vi "elvis_dmm_v2.vi"(0 "Device Name":tag="myDAQ3", 1 "Stop":bool=TRUE, 3 "myDAQ Resistance Input Range (Ohms)":sgl(ring)=200.0 items=["200ohm"=200, "2Kohm"=2000, "20Kohm"=20000, "200Kohm"=200000, "2Mohm"=2000000, "20Mohm"=2e+07], 5 "error in":errorcluster) -> (16 "Measurement":dbl, 17 "Overrange":u16(ring) items=["In Range", "+Over", "-Over", "±Over"], 19 "error out":errorcluster)   [LabVIEW 2013]
doc: "Controls the basic Digital Multimeter capabilities of NI ELVIS II."
uses:
  <vilib>/express/NI ELVISmx/misc.llb/ctl_ProductType.ctl
  <vilib>/DAQmx/read.llb/DAQmx Read (Analog 1D Wfm NChan NSamp).vi
  <vilib>/DAQmx/read.llb/DAQmx Read (Analog DBL 1Chan 1Samp).vi
  <vilib>/DAQmx/create/channels.llb/DAQmx Create Channel (AI-Voltage-Basic).vi
  <vilib>/DAQmx/create/channels.llb/DAQmx Create Channel (AI-Voltage-RMS).vi
  <vilib>/DAQmx/create/channels.llb/DAQmx Create Channel (AI-Current-Basic).vi
  <vilib>/DAQmx/create/channels.llb/DAQmx Create Channel (AI-Current-RMS).vi
  <vilib>/DAQmx/create/channels.llb/DAQmx Create Channel (AI-Resistance).vi
  <vilib>/DAQmx/create/channels.llb/DAQmx Create Channel (AO-FuncGen).vi
  <vilib>/DAQmx/configure/timing.llb/DAQmx Timing (Sample Clock).vi
  <vilib>/measure/matone.llb/Extract Single Tone Information 1 Chan.vi
  <vilib>/DAQmx/miscellaneous.llb/DAQmx Fill In Error Info.vi
  <resource>/objmgr/daqmx.rc
  <vilib>/measure/NI_MAPro.lvlib
panel:
  in  "Measurement":T1(ring)=enum."Resistance"
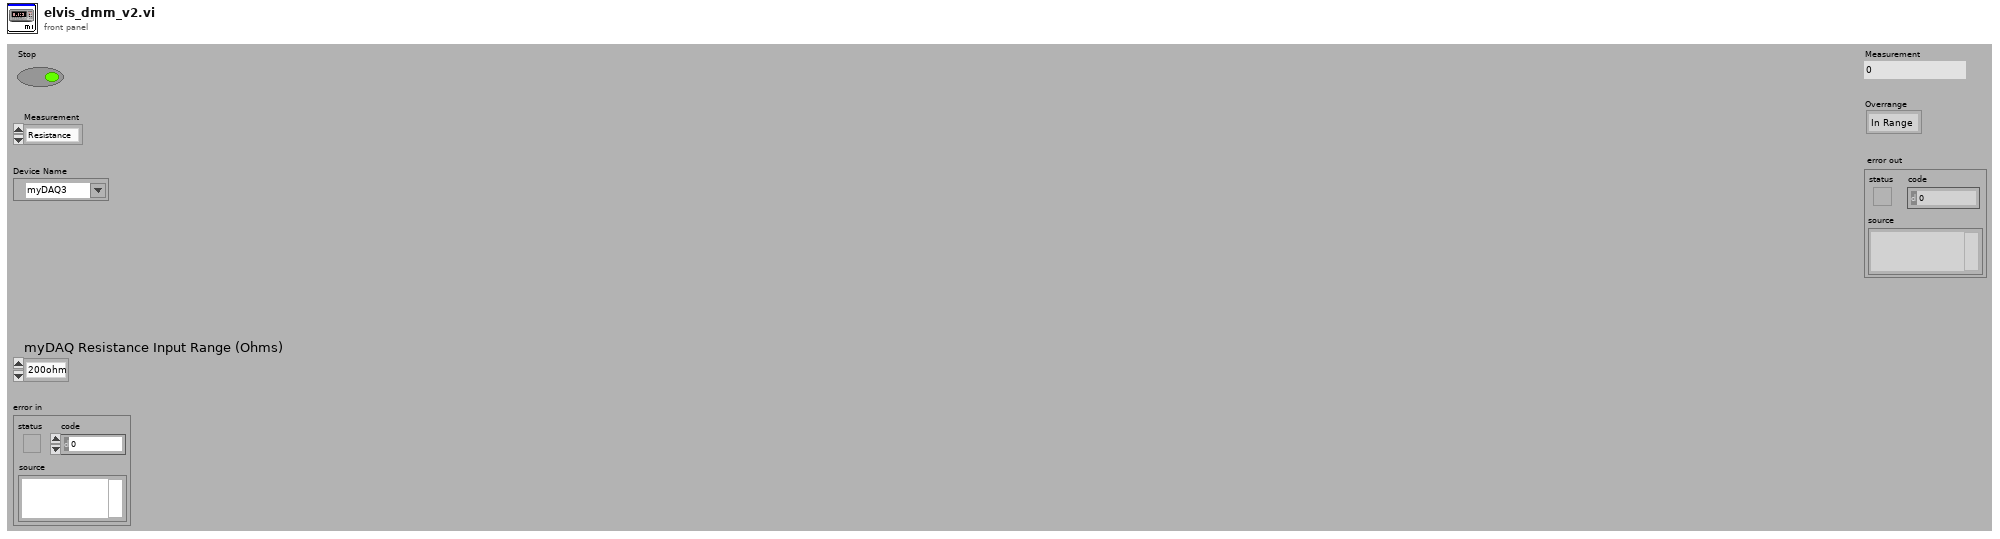
[diagram p1: front panel]
types:
  T1 = enum16{"Volts DC", "Volts AC", "Current DC", "Current AC", "Resistance", "Capacitance", "Inductance", "Diode", "Continuity", "Impedance"}
  T2 = typedef "ctl_ProductType.ctl" = enum16{"NI myDAQ", "NI ELVIS II", "NI ELVIS II+"}
  T3 = cluster{"approx freq. (optional)":dbl, "search (+/- % of Fsampl.)":dbl}
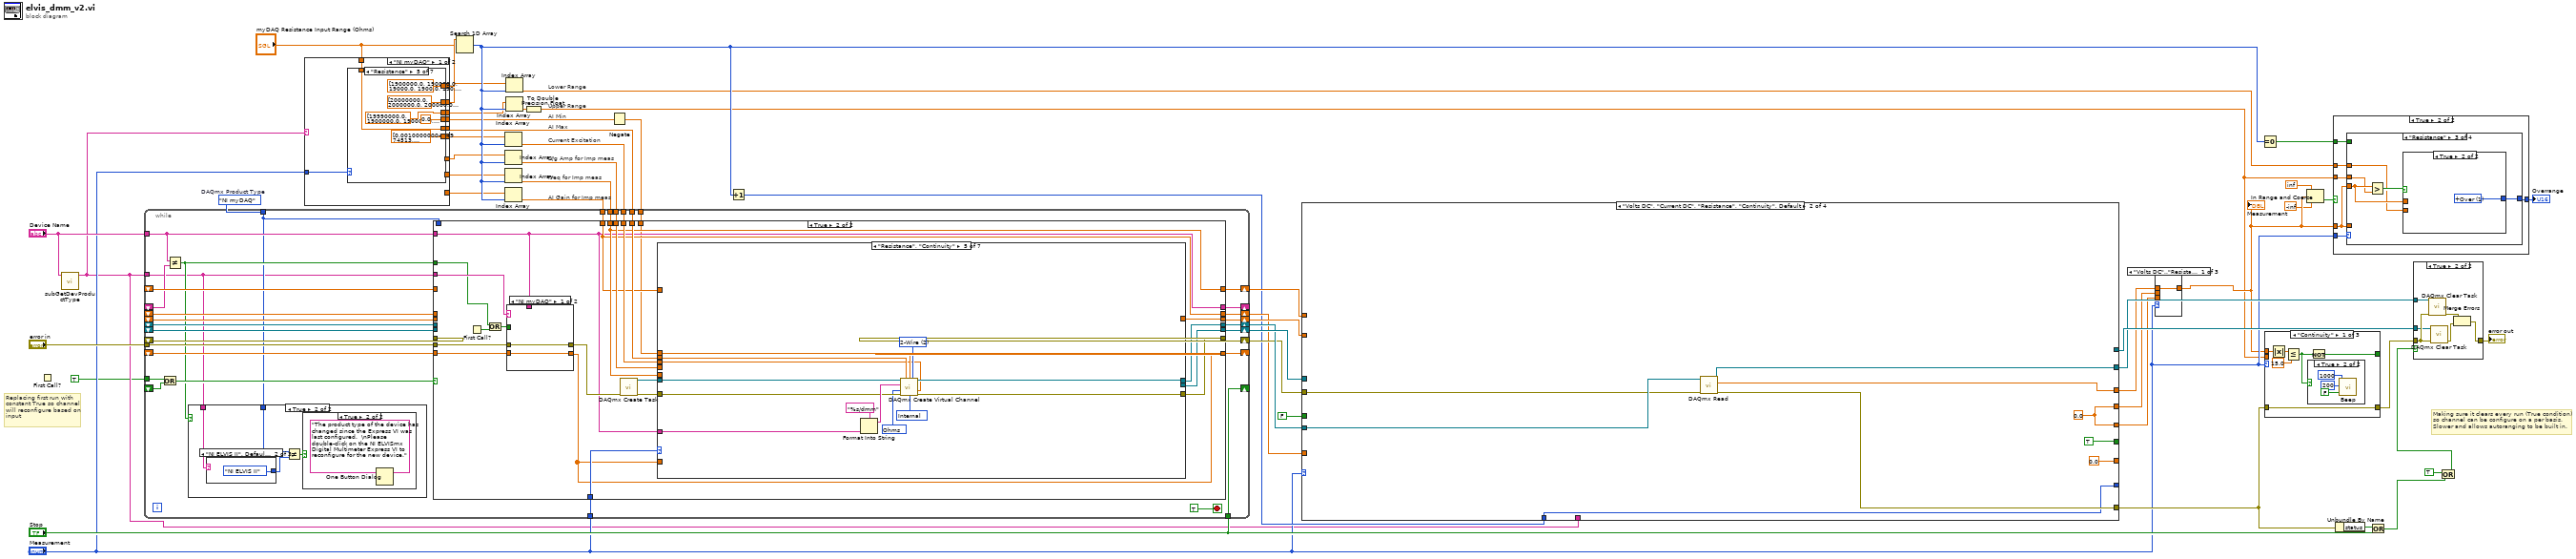
[diagram p0: block diagram]
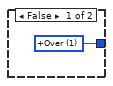
[diagram p2: hidden frame]
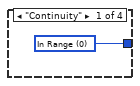
[diagram p3: hidden frame]
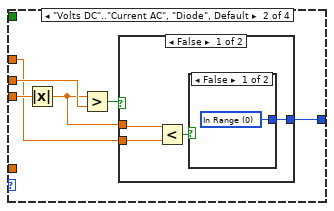
[diagram p4: hidden frame]
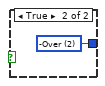
[diagram p5: hidden frame]
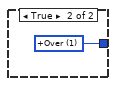
[diagram p6: hidden frame]
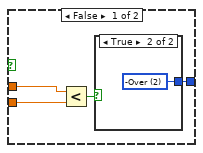
[diagram p7: hidden frame]
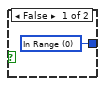
[diagram p8: hidden frame]
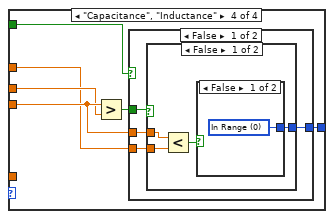
[diagram p9: hidden frame]
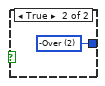
[diagram p10: hidden frame]
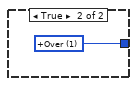
[diagram p11: hidden frame]
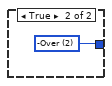
[diagram p12: hidden frame]
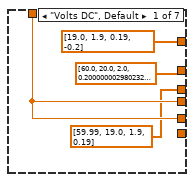
[diagram p13: hidden frame]
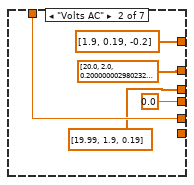
[diagram p14: hidden frame]
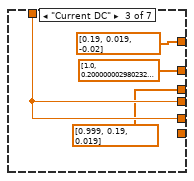
[diagram p15: hidden frame]
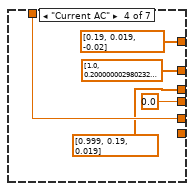
[diagram p16: hidden frame]
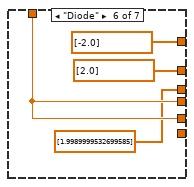
[diagram p17: hidden frame]
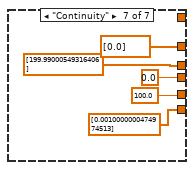
[diagram p18: hidden frame]
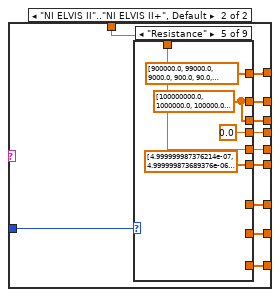
[diagram p19: hidden frame]
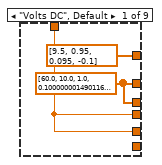
[diagram p20: hidden frame]
diagram:
  w13 = ctl_ProductType."NI myDAQ"  # DAQmx Product Type
  # "Making sure it clears every run (True condition)\nso channel can be configure on a per basis. \nSlower and allows autoranging to be built in."
  # "Replacing first run with \nconstant True so channel\nwill reconfigure based on\ninput"
  # "AI Max"
  # "Lower Range"
  # "Upper Range"
  # "AI Gain for Imp meas"
  # "Freq for Imp meas"
  # "S/g Amp for Imp meas"
  # "AI Min"
  # "Current Excitation"
  n1 = First Call?() -> ()  [unwired: 1 out]
  n2 = call <vilib>:"subGetDevProductType.vi"("activeDevice"="Device Name") -> ("DevProductTypeValue"=w11:string)  [unwired: 9 in, 1 out]
  n3 = case shown="\"NI myDAQ\"" w11 {
    tunnel: [w60 w104] -> w25
    tunnel: [w59 w103] -> w24
    tunnel: [w54 w102] -> w23
    tunnel: [_ w101] -> w22
    tunnel: [_ w100] -> w20
    tunnel: [_ w99] -> w21
    tunnel: "Measurement" -> [w58 w98]
    tunnel: "myDAQ Resistance Input Range (Ohms)" -> [w56 w97]
    tunnel: [w57 w96] -> w15
    tunnel: [w55 w95] -> w16
    tunnel: [w53 w94] -> w12
    frame "NI myDAQ" {
      n4 = case shown="\"Resistance\"" w58 {
        tunnel: [dbl[] [19.0, 1.9, 0.19, -0.2] dbl[] [1.9, 0.19, -0.2] dbl[] [0.19, 0.019, -0.02] dbl[] [0.19, 0.019, -0.02] dbl[] [1900000.0, 190000.0, 19000.0, 1900.0, 190.0, -1000000000.0] sgl[] [-2.0] _] -> w60
        tunnel: [sgl[] [60.0, 20.0, 2.0, 0.2] sgl[] [20.0, 2.0, 0.2] sgl[] [1.0, 0.2, 0.02] sgl[] [1.0, 0.2, 0.02] sgl[] [20000000.0, 2000000.0, 200000.0, 20000.0, 2000.0, 200.0] sgl[] [2.0] sgl[] [0.0]] -> w59
        tunnel: [w62 sgl 0.0 ("Continuity Input Limits (Ohms)") w71 sgl 0.0 ("Continuity Input Limits (Ohms)") sgl 0.0 ("Continuity Input Limits (Ohms)") w88 sgl 0.0 ("Continuity Input Limits (Ohms)")] -> w57
        tunnel: w56 -> [w62 w66 w71 w75 w81 w88 _]
        tunnel: [w62 w66 w71 w75 w81 w88 sgl 100.0 ("Continuity Input Limits (Ohms)")] -> w55
        tunnel: [_ _ _ _ sgl[] [0.001, 0.001, 0.001, 0.001, 0.001, 0.001] _ sgl[] [0.001]] -> w54
        tunnel: [dbl[] [59.99, 19.0, 1.9, 0.19] dbl[] [19.99, 1.9, 0.19] dbl[] [0.999, 0.19, 0.019] dbl[] [0.999, 0.19, 0.019] dbl[] [19990000.0, 1900000.0, 190000.0, 19000.0, 1900.0, 190.0] dbl[] [1.9989999532699585] dbl[] [199.99000549316406]] -> w53
        frame "Volts DC", Default {
        }
        frame "Volts AC" {
        }
        frame "Current DC" {
        }
        frame "Current AC" {
        }
        frame "Resistance" {
        }
        frame "Diode" {
        }
        frame "Continuity" {
        }
      }
    }
    frame "NI ELVIS II".."NI ELVIS II+", Default {
      n5 = case shown="\"Resistance\"" w98 {
        tunnel: [dbl[] [9.5, 0.95, 0.095, -0.1] dbl[] [1.9, 0.19, -0.2] dbl[] [0.0] dbl[] [0.48, -0.5] dbl[] [900000.0, 99000.0, 9000.0, 900.0, 90.0, -1000000000.0] dbl[] [4.9e-05, 9.8e-07, 4.9e-08, 4.9e-09, 4.5e-10, inf] dbl[] [0.01, 0.001, 0.0001] dbl[] [0.95, 0.0] _] -> w104
        tunnel: [w105 w108 w112 w115 w119 w124 w131 w138 w141] -> w103
        tunnel: [_ _ _ _ sgl[] [5e-07, 5e-06, 1e-05, 0.0001, 0.001, 0.001] _ _ _ dbl[] [0.001]] -> w102
        tunnel: [_ _ _ _ _ dbl[] [1.0, 1.0, 1.0, 1.0, 1.0, 1.0] dbl[] [1.0, 0.5, 0.5] _ _] -> w101
        tunnel: [_ _ _ _ _ dbl[] [100.0, 100.0, 1000.0, 1000.0, 1000.0, 10000.0] dbl[] [1000.0, 1000.0, 10000.0] _ _] -> w100
        tunnel: [_ _ _ _ _ dbl[] [10000.0, 10000.0, 10000.0, 100.0, 1.0, 1.0] dbl[] [10000.0, 10000.0, 10000.0] _ _] -> w99
        tunnel: w97 -> [w106 w110 w113 w117 w121 _ _ w139 _]
        tunnel: [w106 sgl 0.0 ("Continuity Input Limits (Ohms)") w113 sgl 0.0 ("Continuity Input Limits (Ohms)") sgl 0.0 ("Continuity Input Limits (Ohms)") w125 w132 w139 0.0 ("Continuity Input Limits (Ohms)")] -> w96
        tunnel: [w106 w110 w113 w117 w121 w125 w132 w139 100.0 ("Continuity Input Limits (Ohms)")] -> w95
        tunnel: [w105 w108 w112 w115 w119 w124 w131 w138 w141] -> w94
        frame "Volts DC", Default {
          w105 = sgl[] [60.0, 10.0, 1.0, 0.1]
        }
        frame "Volts AC" {
          w108 = sgl[] [20.0, 2.0, 0.2]
        }
        frame "Current DC" {
          w112 = sgl[] [2.0]
        }
        frame "Current AC" {
          w115 = sgl[] [2.0, 0.5]
        }
        frame "Resistance" {
          w119 = sgl[] [100000000.0, 1000000.0, 100000.0, 10000.0, 1000.0, 100.0]
        }
        frame "Capacitance" {
          w124 = sgl[] [0.0005, 5e-05, 1e-06, 5e-08, 5e-09, 5e-10]
          n6 = Index Array(array=dbl[] [1.0, 5.0, 5.0, 5.0, 5.0, 5.0]) -> (element=w125:dbl)  [unwired: 1 in]
        }
        frame "Inductance" {
          w131 = sgl[] [0.1, 0.01, 0.001]
          n7 = Index Array(array=dbl[] [1.0, 1.0, 1.0]) -> (element=w132:dbl)  [unwired: 1 in]
        }
        frame "Diode" {
          w138 = sgl[] [10.0, 1.0]
        }
        frame "Continuity" {
          w141 = sgl[] [0.0]
        }
      }
    }
  }
  n8 = Search 1D Array(1D array=w24, element="myDAQ Resistance Input Range (Ohms)") -> (index of element=w27:i32)  [unwired: 1 in]
  n9 = Index Array(array=w23, index=w27) -> (element=w44:dbl)
  n10 = Index Array(array=w22, index=w27) -> (element=w43:dbl)
  n11 = Index Array(array=w20, index=w27) -> (element=w42:dbl)
  n12 = Index Array(array=w21, index=w27) -> (element=w41:dbl)
  n13 = Index Array(array=w12, index=w27) -> (element=w45:dbl)
  n14 = Index Array(array=w25, index=w27) -> (element=w6:dbl)
  n15 = To Double Precision Float(number=w45) -> (double precision float=w5:dbl)
  n16 = Negate(x=w15) -> (-x=w14:dbl)
  n17 = while {
    tunnel: "error in" -> [w177]
    shift-right: [w176] -> w38
    shift-left: _ -> [w174]
    shift-right: [w172] -> _
    shift-left: _ -> [w171]
    tunnel: "Stop" -> [w172]
    tunnel: TRUE ("First Call?: T/F") -> [w169]
    shift-right: [w175] -> w37
    shift-left: _ -> [w168]
    tunnel: "Measurement" -> [w167]
    shift-right: [w166] -> w39
    shift-left: _ -> [w165]
    shift-right: [w164] -> _
    shift-left: _ -> [w148]
    shift-right: [w163] -> w35
    shift-left: _ -> [w162]
    shift-right: [w161] -> _
    shift-left: _ -> [w160]
    shift-right: [w159] -> w36
    shift-left: _ -> [w158]
    shift-right: [w157] -> w40
    shift-left: _ -> [w156]
    tunnel: w11 -> [w145]
    tunnel: w44 -> [w153]
    tunnel: w16 -> [w154]
    tunnel: w43 -> [w152]
    tunnel: w42 -> [w151]
    tunnel: w41 -> [w155]
    tunnel: "Device Name" -> [w149]
    tunnel: w14 -> [w150]
    tunnel: w13 -> [w146]
    stop <- TRUE stop-if-true
    n18 = Or(x=w169, y=w171) -> (x .or. y?=w170:bool)
    n19 = Not Equal?(x=w149, y=w148) -> (x != y?=w147:bool)
    n20 = case shown="True" w147 {
      tunnel: w146 -> [_ w180]
      tunnel: w145 -> [_ w178]
      frame False {
      }
      frame True {
        n21 = case shown="\"NI ELVIS II\", Default" w178 {
          tunnel: [ctl_ProductType."NI ELVIS II+" ("Product Type") ctl_ProductType."NI ELVIS II" ("Product Type") ctl_ProductType."NI myDAQ" ("Product Type")] -> w181
          frame "NI ELVIS II+" {
          }
          frame "NI ELVIS II", Default {
          }
          frame "NI myDAQ" {
          }
        }
        n22 = Not Equal?(x=w180, y=w181) -> (x != y?=w179:bool)
        n23 = case shown="True" w179 {
          frame False {
          }
          frame True {
            n24 = One Button Dialog(message="The product type of the device has changed since the Express VI was last configured.  \nPlease double-click on the NI ELVISmx Digital Multimeter Express VI to reconfigure for the new device.") -> ()  [unwired: 1 in, 1 out]
          }
        }
      }
    }
    n25 = case shown="True" w170 {
      tunnel: w177 -> [_ w215]
      tunnel: [w193 w201] -> w176
      tunnel: [w192 w199] -> w175
      tunnel: w174 -> [w193 _]
      tunnel: w168 -> [w192 _]
      tunnel: w167 -> [_ w208]
      tunnel: [w191 w200] -> w166
      tunnel: w165 -> [w191 _]
      tunnel: [w186 w197] -> w164
      tunnel: [w190 w198] -> w163
      tunnel: w162 -> [w190 _]
      tunnel: [w188 w207] -> w161
      tunnel: w160 -> [w188 w212]
      tunnel: [w189 w203] -> w159
      tunnel: w158 -> [w189 _]
      tunnel: [w187 w202] -> w157
      tunnel: w156 -> [w187 _]
      tunnel: w145 -> [_ w195]
      tunnel: w155 -> [_ w198]
      tunnel: w154 -> [_ w211]
      tunnel: w153 -> [_ w210]
      tunnel: w152 -> [_ w209]
      tunnel: w151 -> [_ w202]
      tunnel: w149 -> [w186 w197]
      tunnel: w150 -> [_ w196]
      tunnel: w146 -> [_ _]
      tunnel: w147 -> [_ w194]
      frame False {
      }
      frame True {
        n26 = First Call?() -> (First Call?: T/F=w214:bool)
        n27 = Or(x=w194, y=w214) -> (x .or. y?=w213:bool)
        n28 = case shown="\"NI myDAQ\"" w195 {
          tunnel: w215 -> [w335 w341]
          tunnel: [w335 w340] -> w206
          tunnel: w213 -> [_ w339]
          tunnel: w197 -> [_ w338]
          tunnel: [w334 w337] -> w207
          tunnel: w212 -> [w334 w336]
          frame "NI myDAQ" {
          }
          frame "NI ELVIS II", Default {
            n29 = case shown="True" w339 {
              tunnel: w341 -> [w343 w347]
              tunnel: [w343 w346] -> w340
              tunnel: w338 -> [_ w345]
              tunnel: [w342 w344] -> w337
              tunnel: w336 -> [w342 _]
              frame False {
              }
              frame True {
                n30 = call <vilib>:"subRecordEEPROMValues.vi"("error in"=w347, "Device Name"=w345) -> ("error out"=w346:errorcluster, "Resistance Array"=w344:sgl[])  [unwired: 8 in]
              }
            }
          }
        }
        n31 = call <vilib>:"DAQmx Create Task.vi"("error in"=w206) -> ("task out"=w204:refnum<k21>, "error out"=w205:errorcluster)  [unwired: 13 in]
        n32 = case shown="\"Resistance\", \"Continuity\"" w208 {
          tunnel: w197 -> [w224 w233 w242 w251 w264 w282 w292]
          tunnel: w204 -> [w221 w230 w239 w248 w261 w279 _]
          tunnel: w205 -> [w220 w229 w238 w247 w260 w278 w290]
          tunnel: [w219 w228 w237 w246 w259 w275 w287] -> w201
          tunnel: [_ _ _ _ _ _ w288] -> w200
          tunnel: [w218 w227 w236 w245 w258 w276 w286] -> w199
          tunnel: w196 -> [w217 w226 w235 w244 w254 w273 w284]
          tunnel: w211 -> [w216 w225 w234 w243 w253 w272 w295]
          tunnel: w210 -> [_ _ _ _ w252 _ _]
          tunnel: [_ _ _ _ _ _ w289] -> w203
          tunnel: w207 -> [_ _ _ _ _ _ w291]
          tunnel: w202 -> [_ _ _ _ _ _ w285]
          tunnel: w209 -> [_ _ _ _ _ _ w293]
          tunnel: w198 -> [_ _ _ _ _ _ w294]
          frame "Volts DC", Default {
            n33 = Format Into String(format string="%s/dmm", w224) -> (resulting string=w222:string)  [unwired: 2 in, 1 out]
            n34 = call-poly <vilib>:"DAQmx Create Virtual Channel.vi"("task in"=w221, "maximum value"=w216, "minimum value"=w217, "physical channels"=w222, "error in"=w220) -> ("task out"=w219:refnum<k21>, "error out"=w218:errorcluster)  [unwired: 9 in]
          }
          frame "Volts AC" {
            n35 = Format Into String(format string="%s/dmm", w233) -> (resulting string=w231:string)  [unwired: 2 in, 1 out]
            n36 = call-poly <vilib>:"DAQmx Create Virtual Channel.vi"("task in"=w230, "maximum value"=w225, "minimum value"=w226, "physical channels"=w231, "error in"=w229) -> ("task out"=w228:refnum<k21>, "error out"=w227:errorcluster)  [unwired: 9 in]
          }
          frame "Current DC" {
            n37 = Format Into String(format string="%s/dmm", w242) -> (resulting string=w240:string)  [unwired: 2 in, 1 out]
            n38 = call-poly <vilib>:"DAQmx Create Virtual Channel.vi"("task in"=w239, "maximum value"=w234, "minimum value"=w235, "physical channels"=w240, "error in"=w238) -> ("task out"=w237:refnum<k21>, "error out"=w236:errorcluster)  [unwired: 9 in]
          }
          frame "Current AC" {
            n39 = Format Into String(format string="%s/dmm", w251) -> (resulting string=w249:string)  [unwired: 2 in, 1 out]
            n40 = call-poly <vilib>:"DAQmx Create Virtual Channel.vi"("task in"=w248, "maximum value"=w243, "minimum value"=w244, "physical channels"=w249, "error in"=w247) -> ("task out"=w246:refnum<k21>, "error out"=w245:errorcluster)  [unwired: 9 in]
          }
          frame "Resistance", "Continuity" {
            w255 = 2 items=["2-Wire"=2, "3-Wire"=3, "4-Wire"=4] ("resistance configuration")
            w256 = 10384 items=["Ohms"=10384, "From Custom Scale"=10065] ("units")
            w257 = 10200 items=["Internal"=10200, "External"=10167, "None"=10230] ("current excitation source")
            n41 = Format Into String(format string="%s/dmm", w264) -> (resulting string=w262:string)  [unwired: 2 in, 1 out]
            n42 = call-poly <vilib>:"DAQmx Create Virtual Channel.vi"("task in"=w261, "maximum value"=w253, "minimum value"=w254, "resistance configuration"=w255, "physical channels"=w262, "units"=w256, "current excitation value"=w252, "error in"=w260, "current excitation source"=w257) -> ("task out"=w259:refnum<k21>, "error out"=w258:errorcluster)  [unwired: 5 in]
          }
          frame "Diode" {
            w274 = 10200 items=["Internal"=10200, "External"=10167, "None"=10230] ("AI.Excit.Src")
            n43 = Format Into String(format string="%s/dmm", w282) -> (resulting string=w277:string)  [unwired: 2 in, 1 out]
            n44 = call-poly <vilib>:"DAQmx Create Virtual Channel.vi"("task in"=w279, "maximum value"=w272, "minimum value"=w273, "physical channels"=w277, "error in"=w278) -> ("task out"=w280:refnum<k21>, "error out"=w281:errorcluster)  [unwired: 9 in]
            n45 = Equal?(x=w272, y=10.0) -> (x = y?=w270:bool)
            n46 = Select(t=0.0001, s=w270, f=0.001) -> (s? t:f=w267:dbl)
            n47 = property class="DAQmx Channel"(reference=w280, error in=w281, "AI.Excit.Src"=w274, "AI.Excit.Val"=w267) -> (reference out=w265:refnum<k21>, error out=w266:errorcluster)
            n48 = call <vilib>:"DAQmx Start Task.vi"("task/channels in"=w265, "error in"=w266) -> ("task out"=w275:refnum<k21>, "error out"=w276:errorcluster)  [unwired: 12 in]
          }
          frame "Capacitance", "Inductance" {
            w302 = 10178 items=["Finite Samples"=10178, "Continuous Samples"=10123, "Hardware Timed Single Point"=12522] ("sample mode")
            w296 = 14751 items=["Sine"=14751, "Triangle"=14752, "Square"=14753, "Sawtooth"=14754] ("type")
            n49 = Format Into String(format string="%s/_DUTPos", w292) -> (resulting string=w306:string)  [unwired: 2 in, 1 out]
            n50 = Format Into String(format string="%s/_DUTNeg", w292) -> (resulting string=w305:string)  [unwired: 2 in, 1 out]
            n51 = Format Into String(format string="%s/_fgenImpedance", w292) -> (resulting string=w297:string)  [unwired: 2 in, 1 out]
            n52 = call <vilib>:"DAQmx Create Task.vi"("error in"=w290) -> ("task out"=w299:refnum<k21>, "error out"=w298:errorcluster)  [unwired: 13 in]
            n53 = Build Array(w306, w305) -> (w304:string[])
            n54 = call-poly <vilib>:"DAQmx Create Virtual Channel.vi"("task in"=w299, "frequency"=w285, "amplitude"=w293, "physical channels"=w297, "type"=w296, "error in"=w298) -> ("task out"=w288:refnum<k21>, "error out"=w314:errorcluster)  [unwired: 8 in]
            n55 = case shown="10000, Default" w294 {
              tunnel: [2 ("index") 1 ("index") 0 ("index")] -> w313
              frame 10000, Default {
              }
              frame 100 {
              }
              frame 1 {
              }
            }
            n56 = call <vilib>:"DAQmx Create Task.vi"("error in"=w314) -> ("task out"=w303:refnum<k21>, "error out"=w301:errorcluster)  [unwired: 13 in]
            n57 = Index Array(array=w291, index=w313) -> (element=w289:sgl)
            n58 = for {
              tunnel: w304 -> [w330] mode=indexing
              shift-right: [w328] -> w310
              shift-left: w301 -> [w331]
              shift-right: [w329] -> w312
              shift-left: w303 -> [w332]
              tunnel: w295 -> [w327]
              tunnel: w284 -> [w326]
              w333 = 10083 items=["default"=-1, "RSE"=10083, "NRSE"=10078, "Differential"=10106, "Pseudodifferential"=12529] ("input terminal configuration")
              n59 = call-poly <vilib>:"DAQmx Create Virtual Channel.vi"("task in"=w332, "maximum value"=w327, "minimum value"=w326, "input terminal configuration"=w333, "physical channels"=w330, "error in"=w331) -> ("task out"=w329:refnum<k21>, "error out"=w328:errorcluster)  [unwired: 8 in]
            }
            n60 = property class="DAQmx Channel"(reference=w312, error in=w310, "AI.Gain"=w294) -> (reference out=w309:refnum<k21>, error out=w311:errorcluster)
            n61 = Greater?(x=w285, y=200.0) -> (0:w316:bool)
            n62 = case shown="False" w316 {
              tunnel: [25000 ("samples per channel") 250000 ("samples per channel")] -> w318
              tunnel: [50000.0 ("rate") 500000.0 ("rate")] -> w317
              frame False {
              }
              frame True {
              }
            }
            n63 = call-poly <vilib>:"DAQmx Timing.vi"("task/channels in"=w309, "sample mode"=w302, "samples per channel"=w318, "rate"=w317, "error in"=w311) -> ("task out"=w287:refnum<k21>, "error out"=w286:errorcluster)  [unwired: 9 in]
          }
        }
      }
    }
  }
  n64 = Increment(x=w27) -> (x+1=w26:i32)
  n65 = case shown="\"Volts DC\", \"Current DC\", \"Resistance\", \"Continuity\", Default" "Measurement" {
    selector: "Measurement" -> [w360 _ _ _]
    tunnel: w39 -> [w405 _ _ _]
    tunnel: w37 -> [w404 w477 w491 w542]
    tunnel: w38 -> [w394 w478 w492 w543]
    tunnel: w35 -> [w393 _ _ _]
    tunnel: [w403 _ _ _] -> w33
    tunnel: [w402 w475 w486 w536] -> w32
    tunnel: [w348 w474 w484 w538] -> w28
    tunnel: [0.0 ("data") w476 w485 w537] -> w31
    tunnel: [w351 w479 w493 w544] -> w30
    tunnel: [w352 w479 w493 w544] -> w29
    tunnel: w36 -> [w356 _ _ _]
    tunnel: [w353 0.0 ("Computed Value") 0.0 ("Computed Value") 0.0 ("Computed Value")] -> _
    tunnel: FALSE ("Run Once?") -> [w355 _ w487 _]
    tunnel: [w349 w472 w489 w540] -> _
    tunnel: w26 -> [w354 w472 w489 w540]
    tunnel: [w350 TRUE ("Good Range?") TRUE ("Good Range?") TRUE ("Good Range?")] -> _
    tunnel: w40 -> [w357 _ _ _]
    tunnel: w11 -> [_ _ w480 _]
    frame "Capacitance", "Inductance" {
      n66 = call <vilib>:"DAQmx Start Task.vi"("task/channels in"=w405, "error in"=w404) -> ("task out"=w399:refnum<k21>, "error out"=w400:errorcluster)  [unwired: 12 in]
      n67 = call <vilib>:"DAQmx Stop Task.vi"("task/channels in"=w399, "error in"=w400) -> ("task out"=w403:refnum<k21>, "error out"=w396:errorcluster)  [unwired: 12 in]
      n68 = property class="DAQmx Channel"(reference=w394, error in=w396, "AI.Gain"=w393) -> (reference out=w397:refnum<k21>, error out=w395:errorcluster)
      n69 = call-poly <vilib>:"DAQmx Read.vi"("task/channels in"=w397, "error in"=w395) -> ("task out"=w402:refnum<k21>, "data"=w398:waveform(dbl)[], "error out"=w348:errorcluster)  [unwired: 11 in]
      n70 = Index Array(array=w398) -> (element #1=w359:waveform(dbl), element #2=w392:waveform(dbl))  [unwired: 2 in]
      n71 = Negate(x=w392) -> (-x=w358:waveform(dbl))
      n72 = Bundle By Name(cluster=T3 {"approx freq. (optional)"=-1.0, "search (+/- % of Fsampl.)"=5.0} ("advanced search"), "approx freq. (optional)"=w357, "search (+/- % of Fsampl.)"=1.0) -> (w361:T3)
      n73 = call-poly <vilib>:"Extract Single Tone Information.vi"("advanced search"=w361, "time signal in"=w359) -> ("detected phase (deg)"=w385:dbl, "detected amplitude"=w387:dbl, "detected frequency"=w389:dbl)  [unwired: 4 in, 3 out]
      n74 = call-poly <vilib>:"Extract Single Tone Information.vi"("advanced search"=w361, "time signal in"=w358) -> ("detected phase (deg)"=w384:dbl, "detected amplitude"=w391:dbl)  [unwired: 4 in, 4 out]
      n75 = Divide(x=w391, y=w356) -> (x/y=w388:dbl)
      n76 = Divide(x=w387, y=w388) -> (x/y=w386:dbl)
      n77 = Subtract(x=w385, y=w384) -> (x-y=w367:dbl)
      n78 = case shown="True" w355 {
        tunnel: w354 -> [w407 w411]
        tunnel: w391 -> [_ w412]
        tunnel: [w407 w410] -> w349
        tunnel: [TRUE w409] -> w350
        tunnel: w360 -> [_ w408]
        frame False {
        }
        frame True {
          n79 = Greater?(x=w412, y=4.2) -> (0:w413:bool)
          n80 = case shown="True" w413 {
            tunnel: w412 -> [w421 _]
            tunnel: w411 -> [w418 w441]
            tunnel: [w417 w442] -> w410
            tunnel: [w416 FALSE] -> w409
            tunnel: w408 -> [w415 _]
            frame False {
              n81 = Less?(x=w421, y=0.001) -> (x < y?=w419:bool)
              n82 = case shown="True" w419 {
                tunnel: w418 -> [w423 w426]
                tunnel: [w423 w425] -> w417
                tunnel: [TRUE FALSE] -> w416
                tunnel: w415 -> [_ w424]
                frame False {
                }
                frame True {
                  n83 = case shown="Default" w424 {
                    tunnel: w426 -> [w429 w433 w438]
                    tunnel: [w428 w433 w436] -> w425
                    frame "Inductance" {
                      w430 = 3 ("y")
                      n84 = Equal?(x=w430, y=w429) -> (x = y?=w432:bool)
                      n85 = Increment(x=w429) -> (x+1=w431:i32)
                      n86 = Select(t=w430, s=w432, f=w431) -> (s? t:f=w428:i32)
                    }
                    frame Default {
                    }
                    frame "Capacitance" {
                      w434 = 6 ("y")
                      n87 = Equal?(x=w434, y=w438) -> (x = y?=w437:bool)
                      n88 = Increment(x=w438) -> (x+1=w435:i32)
                      n89 = Select(t=w434, s=w437, f=w435) -> (s? t:f=w436:i32)
                    }
                  }
                }
              }
            }
            frame True {
              w439 = 1 ("x")
              n90 = Equal?(x=w439, y=w441) -> (x = y?=w443:bool)
              n91 = Decrement(x=w441) -> (x-1=w440:i32)
              n92 = Select(t=w439, s=w443, f=w440) -> (s? t:f=w442:i32)
            }
          }
        }
      }
      n93 = Subtract(x=w367, y=360.0) -> (x-y=w380:dbl)
      n94 = Greater?(x=w367, y=180.0) -> (0:w382:bool)
      n95 = Select(t=w380, s=w382, f=w367) -> (s? t:f=w375:dbl)
      n96 = Add(x=w367, y=360.0) -> (x+y=w376:dbl)
      n97 = Less?(x=w375, y=-180.0) -> (x < y?=w378:bool)
      n98 = Select(t=w376, s=w378, f=w375) -> (s? t:f=w366:dbl)
      n99 = In Range and Coerce(upper limit=90.0, x=w366, lower limit=-90.0) -> (coerced(x)=w365:dbl)  [unwired: 1 out]
      n100 = Divide(x=3.141592653589793 ("Pi"), y=180.0) -> (x/y=w372:dbl)
      n101 = Multiply(x=w365, y=w372) -> (x*y=w371:dbl)
      n102 = Sine(x=w371) -> (sin(x)=w370:dbl)
      n103 = Multiply(x=w386, y=w370) -> (x*y=w390:dbl)
      n104 = Less Than 0?(x=w390) -> (x < 0?=w364:bool)
      n105 = case shown="\"Capacitance\"" w360 {
        tunnel: w389 -> [w447 _ w452]
        tunnel: w390 -> [w446 _ w451]
        tunnel: [w445 _ w450] -> w353
        frame "Inductance" {
          n106 = Multiply(x=6.283185307179586 ("Pi Multiplied By 2"), y=w447) -> (x*y=w449:dbl)
          n107 = Divide(x=w446, y=w449) -> (x/y=w445:dbl)
        }
        frame Default {
        }
        frame "Capacitance" {
          n108 = Multiply(x=6.283185307179586 ("Pi Multiplied By 2"), y=w452) -> (x*y=w455:dbl)
          n109 = Negate(x=w451) -> (-x=w454:dbl)
          n110 = Multiply(x=w455, y=w454) -> (x*y=w456:dbl)
          n111 = Reciprocal(x=w456) -> (1/x=w450:dbl)
        }
      }
      n112 = case shown="True" w364 {
        tunnel: w389 -> [w460 w469]
        tunnel: w390 -> [w459 w465]
        tunnel: [w458 inf ("Positive Infinity")] -> w351
        tunnel: [inf ("Positive Infinity") w468] -> w352
        frame True {
          n113 = Multiply(x=6.283185307179586 ("Pi Multiplied By 2"), y=w460) -> (x*y=w463:dbl)
          n114 = Negate(x=w459) -> (-x=w462:dbl)
          n115 = Multiply(x=w463, y=w462) -> (x*y=w464:dbl)
          n116 = Reciprocal(x=w464) -> (1/x=w458:dbl)
        }
        frame False {
          n117 = Multiply(x=6.283185307179586 ("Pi Multiplied By 2"), y=w469) -> (x*y=w466:dbl)
          n118 = Divide(x=w465, y=w466) -> (x/y=w468:dbl)
        }
      }
    }
    frame "Volts DC", "Current DC", "Resistance", "Continuity", Default {
      w479 = 0.0 ("Phase")
      n119 = call-poly <vilib>:"DAQmx Read.vi"("task/channels in"=w478, "error in"=w477) -> ("task out"=w475:refnum<k21>, "data"=w476:dbl, "error out"=w474:errorcluster)  [unwired: 11 in]
    }
    frame "Volts AC", "Current AC" {
      w493 = 0.0 ("Phase")
      n120 = call-poly <vilib>:"DAQmx Read.vi"("task/channels in"=w492, "error in"=w491) -> ("task out"=w483:refnum<k21>, "data"=w482:dbl, "error out"=w481:errorcluster)  [unwired: 11 in]
      n121 = case shown="\"NI ELVIS II\", Default" w480 {
        tunnel: w487 -> [_ w505]
        tunnel: [w495 w504] -> w486
        tunnel: [w496 w503] -> w485
        tunnel: [w494 w502] -> w484
        tunnel: w483 -> [w495 w501]
        tunnel: w482 -> [w496 w500]
        tunnel: w481 -> [w494 w499]
        frame "NI myDAQ" {
          # "No need to add the delay or to discard the initial readings for myDAQ."
        }
        frame "NI ELVIS II", Default {
          # "This is a workaround for the issue with ELVIS II/II+ AC measurements"
          n122 = Build Array(w505, TRUE ("Run Once?")) -> (w506:bool[])
          n123 = Boolean Array To Number(Boolean array=w506) -> (number=w498:u32)
          n124 = case shown="2" w498 {
            tunnel: w500 -> [w508 _ _]
            tunnel: w501 -> [w507 w515 w527]
            tunnel: w499 -> [w509 w514 w524]
            tunnel: [w509 w513 w523] -> w502
            tunnel: [w508 w512 w525] -> w503
            tunnel: [w507 w511 w526] -> w504
            frame 0, Default {
              # "Specific Range, Run Continuous"
            }
            frame 1, 3 {
              # "Auto Range, Run Continuous/Run Once"
              n125 = for {
                N: 3 -> [_]
                tunnel: w515 -> [w520]
                tunnel: w514 -> [w519]
                tunnel: [w518] -> w513
                tunnel: [w517] -> w512
                tunnel: [w516] -> w511
                n126 = call-poly <vilib>:"DAQmx Read.vi"("task/channels in"=w520, "error in"=w519) -> ("task out"=w516:refnum<k21>, "data"=w517:dbl, "error out"=w518:errorcluster)  [unwired: 11 in]
              }
            }
            frame 2 {
              # "Specific Range, Run Once"
              n127 = flat-sequence {
                tunnel: w524 -> [w529]
                tunnel: w527 -> [w530]
                tunnel: [w530] -> w522
                tunnel: [w529] -> w521
                tunnel: [w533] -> w526
                tunnel: [w531] -> w525
                tunnel: [w532] -> w523
                tunnel: w522 -> [w535]
                tunnel: w521 -> [w534]
                tunnel: [w531] -> _
                frame #0 {
                  n128 = Wait Until Next ms Multiple(millisecond multiple=u32 5000) -> ()  [unwired: 1 out]
                }
                frame #1 {
                  n129 = call-poly <vilib>:"DAQmx Read.vi"("task/channels in"=w535, "error in"=w534) -> ("task out"=w533:refnum<k21>, "data"=w531:dbl, "error out"=w532:errorcluster)  [unwired: 11 in]
                }
              }
            }
          }
        }
      }
    }
    frame "Diode" {
      w544 = 0.0 ("Phase")
      n130 = call-poly <vilib>:"DAQmx Read.vi"("task/channels in"=w543, "error in"=w542) -> ("task out"=w536:refnum<k21>, "data"=w537:dbl, "error out"=w538:errorcluster)  [unwired: 11 in]
    }
  }
  n131 = case shown="\"Volts DC\"..\"Resistance\", \"Diode\", \"Continuity\", Default" "Measurement" {
    tunnel: w31 -> [w545 _ _]
    tunnel: w30 -> [_ w546 _]
    tunnel: w29 -> [_ _ w547]
    tunnel: [w545 w546 w547] -> w10
    frame "Volts DC".."Resistance", "Diode", "Continuity", Default {
    }
    frame "Capacitance" {
    }
    frame "Inductance" {
    }
  }
  "Measurement" <- w10
  n132 = Equal To 0?(x=w27) -> (x = 0?=w46:bool)
  n133 = case shown="\"Continuity\"" "Measurement" {
    tunnel: w10 -> [w553 _ w562]
    tunnel: w28 -> [w552 w557 w561]
    tunnel: [w552 w557 w561] -> w48
    tunnel: [w548 _ w559] -> _
    tunnel: w5 -> [_ _ w558]
    frame "Continuity" {
      n134 = Absolute Value(x=w553) -> (abs(x)=w550:dbl)
      n135 = Less Or Equal?(x=w550, y=15.0) -> (x <= y?=w549:bool)
      n136 = case shown="True" w549 {
        frame False {
        }
        frame True {
          n137 = call <vilib>:"Beep.vi"("use system alert? (T)"=FALSE, "duration (msec)"=u32 200, "frequency (Hz)"=u32 1000) -> ()  [unwired: 9 in]
        }
      }
      n138 = Not(x=w549) -> (.not. x?=w548:bool)
    }
    frame Default {
    }
    frame "Diode" {
      n139 = Less Or Equal?(x=w562, y=w558) -> (x <= y?=w560:bool)
      n140 = Not(x=w560) -> (.not. x?=w559:bool)
    }
  }
  n141 = In Range and Coerce(upper limit=inf ("Positive Infinity"), x=w10, lower limit=-inf ("Negative Infinity")) -> (In Range?=w7:bool)  [unwired: 1 out]
  n142 = case shown="True" w7 {
    tunnel: w10 -> [_ w569]
    tunnel: [w563 w568] -> w47
    tunnel: w46 -> [_ w567]
    tunnel: w6 -> [_ w566]
    tunnel: "Measurement" -> [_ w565]
    tunnel: w5 -> [_ w564]
    frame False {
      w563 = u16 1 items=["In Range", "+Over", "-Over", "±Over"] ("Overrange")
    }
    frame True {
      n143 = case shown="\"Resistance\"" w565 {
        tunnel: w569 -> [_ _ _ _]
        tunnel: w569 -> [_ w573 w586 w599]
        tunnel: [w570 w575 w587 w600] -> w568
        tunnel: w564 -> [_ w574 w585 w598]
        tunnel: w566 -> [_ w571 w584 w597]
        tunnel: w567 -> [_ _ _ w596]
        frame "Continuity" {
          w570 = u16 0 items=["In Range", "+Over", "-Over", "±Over"] ("Overrange")
        }
        frame "Volts DC".."Current AC", "Diode", Default {
          n144 = Absolute Value(x=w573) -> (abs(x)=w572:dbl)
          n145 = Greater?(x=w572, y=w574) -> (0:w576:bool)
          n146 = case shown="False" w576 {
            tunnel: w571 -> [w580 _]
            tunnel: w572 -> [w579 _]
            tunnel: [w577 w583] -> w575
            frame False {
              n147 = Less?(x=w579, y=w580) -> (x < y?=w578:bool)
              n148 = case shown="False" w578 {
                tunnel: [w581 w582] -> w577
                frame False {
                  w581 = u16 0 items=["In Range", "+Over", "-Over", "±Over"] ("Overrange")
                }
                frame True {
                  w582 = u16 2 items=["In Range", "+Over", "-Over", "±Over"] ("Overrange")
                }
              }
            }
            frame True {
              w583 = u16 1 items=["In Range", "+Over", "-Over", "±Over"] ("Overrange")
            }
          }
        }
        frame "Resistance" {
          n149 = Greater?(x=w586, y=w585) -> (0:w588:bool)
          n150 = case shown="True" w588 {
            tunnel: w584 -> [w592 _]
            tunnel: w586 -> [w591 _]
            tunnel: [w589 w595] -> w587
            frame False {
              n151 = Less?(x=w591, y=w592) -> (x < y?=w590:bool)
              n152 = case shown="True" w590 {
                tunnel: [w593 w594] -> w589
                frame False {
                  w593 = u16 0 items=["In Range", "+Over", "-Over", "±Over"] ("Overrange")
                }
                frame True {
                  w594 = u16 2 items=["In Range", "+Over", "-Over", "±Over"] ("Overrange")
                }
              }
            }
            frame True {
              w595 = u16 1 items=["In Range", "+Over", "-Over", "±Over"] ("Overrange")
            }
          }
        }
        frame "Capacitance", "Inductance" {
          n153 = Greater?(x=w599, y=w598) -> (0:w601:bool)
          n154 = case shown="False" w596 {
            tunnel: w601 -> [w605 _]
            tunnel: [w604 w613] -> w600
            tunnel: w599 -> [w603 _]
            tunnel: w597 -> [w602 _]
            frame False {
              n155 = case shown="False" w605 {
                tunnel: w602 -> [w609 _]
                tunnel: w603 -> [w608 _]
                tunnel: [w606 w612] -> w604
                frame False {
                  n156 = Less?(x=w608, y=w609) -> (x < y?=w607:bool)
                  n157 = case shown="False" w607 {
                    tunnel: [w610 w611] -> w606
                    frame False {
                      w610 = u16 0 items=["In Range", "+Over", "-Over", "±Over"] ("Overrange")
                    }
                    frame True {
                      w611 = u16 2 items=["In Range", "+Over", "-Over", "±Over"] ("Overrange")
                    }
                  }
                }
                frame True {
                  w612 = u16 1 items=["In Range", "+Over", "-Over", "±Over"] ("Overrange")
                }
              }
            }
            frame True {
              w613 = u16 2 items=["In Range", "+Over", "-Over", "±Over"] ("Overrange")
            }
          }
        }
      }
    }
  }
  "Overrange" <- w47
  n158 = Unbundle By Name(w28) -> ("status"=w50:bool)
  n159 = Or(x=w50, y="Stop") -> (x .or. y?=w3:bool)
  n160 = Or(x=TRUE, y=w3) -> (x .or. y?=w2:bool)
  n161 = case shown="True" w2 {
    tunnel: [w614 w618] -> w51
    tunnel: w48 -> [w614 w617]
    tunnel: w32 -> [_ w616]
    tunnel: w33 -> [_ w615]
    frame False {
    }
    frame True {
      n162 = call <vilib>:"DAQmx Clear Task.vi"("task in"=w616, "error in"=w617) -> ("error out"=w620:errorcluster)  [unwired: 13 in]
      n163 = call <vilib>:"DAQmx Clear Task.vi"("task in"=w615, "error in"=w617) -> ("error out"=w619:errorcluster)  [unwired: 13 in]
      n164 = Merge Errors(w620, w619) -> (w618:errorcluster)
    }
  }
  "error out" <- w51
